vi "DISPLAY  LabPanel Data file V1.1 (2).vi"() -> ()   [LabVIEW 2013]
panel:
  in  "Open selected file":bool
  out "file error":errorcluster
  in  "Select  LabPanel TDMS data file to view":path
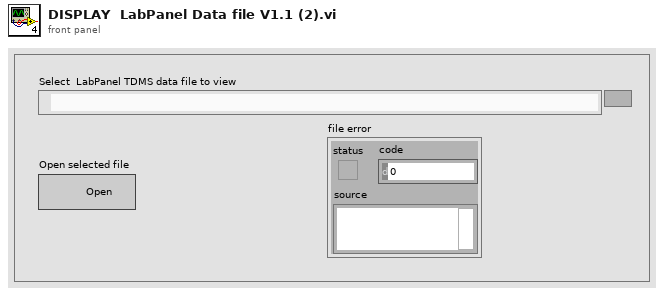
[diagram p1: front panel]
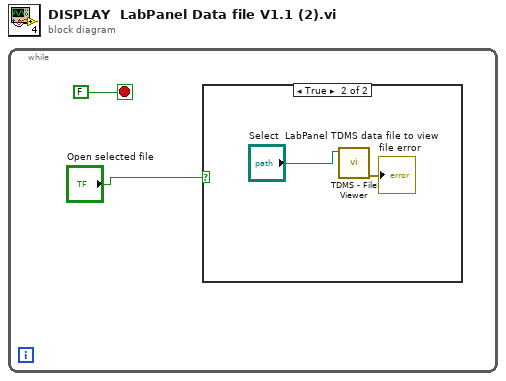
[diagram p0: block diagram]
diagram:
  n1 = while {
    stop <- FALSE stop-if-true
    n2 = case shown="True" "Open selected file" {
      frame False {
      }
      frame True {
        n3 = call <vilib>:"TDMS - File Viewer.vi"("file path"="Select  LabPanel TDMS data file to view") -> ("error out"=→"file error":errorcluster)  [unwired: 5 in, 1 out]
      }
    }
  }
